vi "abort_camera.vi"() -> ()   [LabVIEW 2012]
panel:
  out "Camera Error":errorcluster
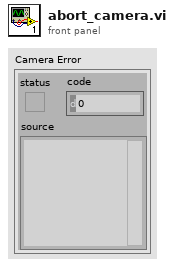
[diagram p1: front panel]
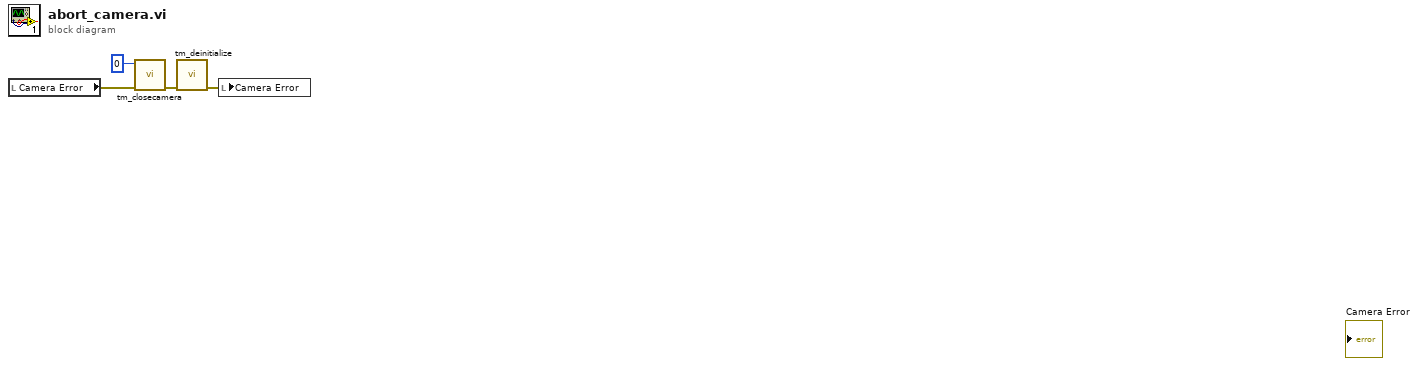
[diagram p0: block diagram]
diagram:
  n1 = local read "Camera Error"() -> (w3:errorcluster)
  n2 = call <userlib>:"tm_closecamera.vi"("error in (no error)"=w3, "Handle in"=u32 0) -> ("error out"=w1:errorcluster)  [unwired: 9 in]
  n3 = call <userlib>:"tm_deinitialize.vi"("error in (no error)"=w1) -> ("error out"=w4:errorcluster)  [unwired: 10 in]
  n4 = local write "Camera Error"(w4) -> ()
